vi "Run.vi"(8 "Column":i32, 9 "Row":i32, 10 "Maze (0: Empty, -1: Enemy. 1: Teammate)":i32[](array[numeric]), 11 "Line Dancer in":refnum<class "Brick Wall.lvclass">) -> (0 "Replicated":refnum<class "Square.lvclass">, 1 "Direction":T1, 2 "Action":T2, 3 "Line Dancer out":refnum<class "Brick Wall.lvclass">)   [LabVIEW 2015, in "Brick Wall.lvclass"]
uses:
  Brick Wall.lvclass
  Type Defs/Action Enum.ctl
  Type Defs/Direction Enum.ctl
  Square/Square.lvclass
  Common/Position.ctl
  Brick Wall.lvclass/Brick Wall.ctl
  Brick Wall Type.ctl
  SubVIs/Read-Only Globals.vi
  Common/Reverse Direction.vi
  Type Defs/SB Type Defs.lvlib
  Common/Common.lvlib
panel:
  # "NW\nN\nNE\nE\nSE\nS\nSW\nW"
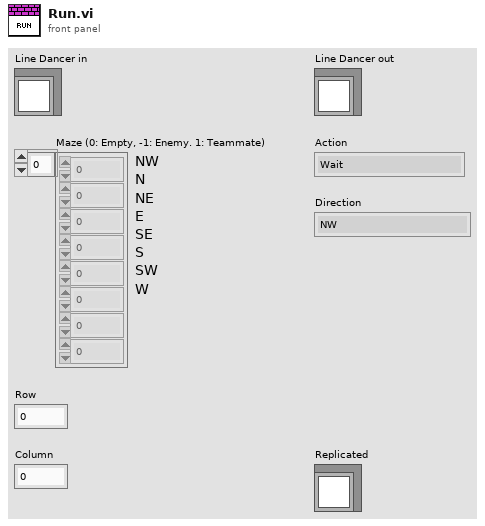
[diagram p1: front panel]
types:
  T1 = typedef "SB Type Defs.lvlib/Direction Enum.ctl" = enum16{"NW", "N", "NE", "E", "SE", "S", "SW", "W"}
  T2 = typedef "SB Type Defs.lvlib/Action Enum.ctl" = enum16{"Wait", "Move", "Attack", "Replicate"}
  T3 = typedef "Common.lvlib/Position.ctl" = cluster{"Column":i32, "Row":i32}
  T4 = typedef "Brick Wall.lvclass/Brick Wall Type.ctl" = enum16{"Row Starter", "Mover", "Starter", "Spawner", "Mason", "Wall"}
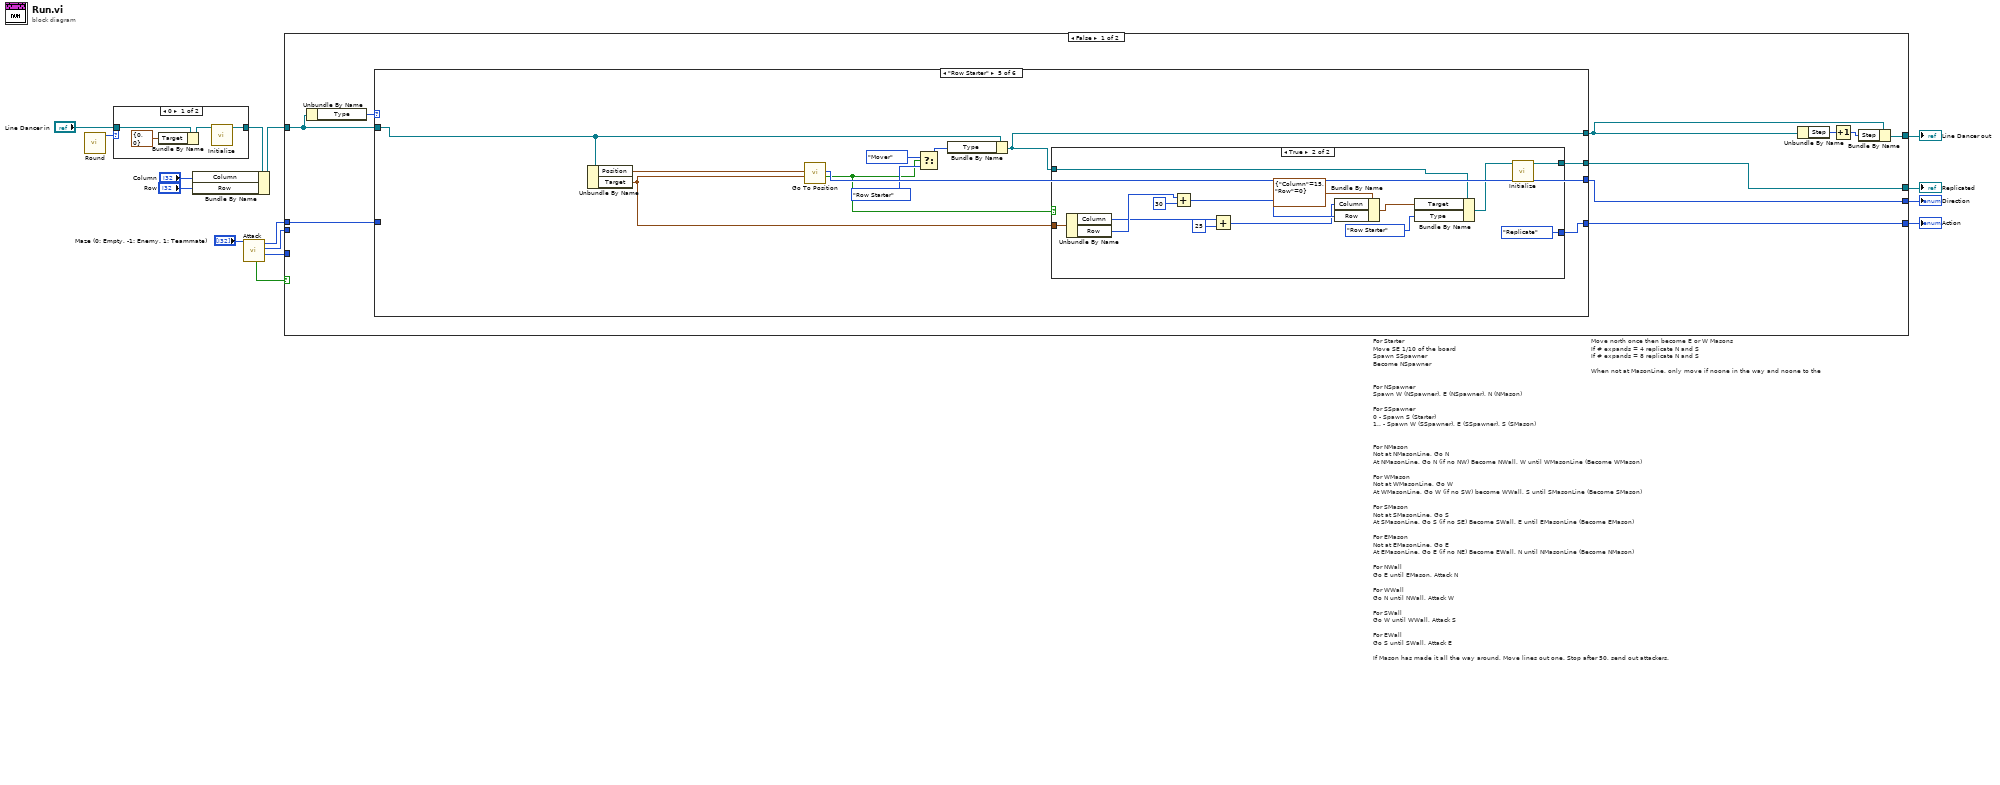
[diagram p0: block diagram]
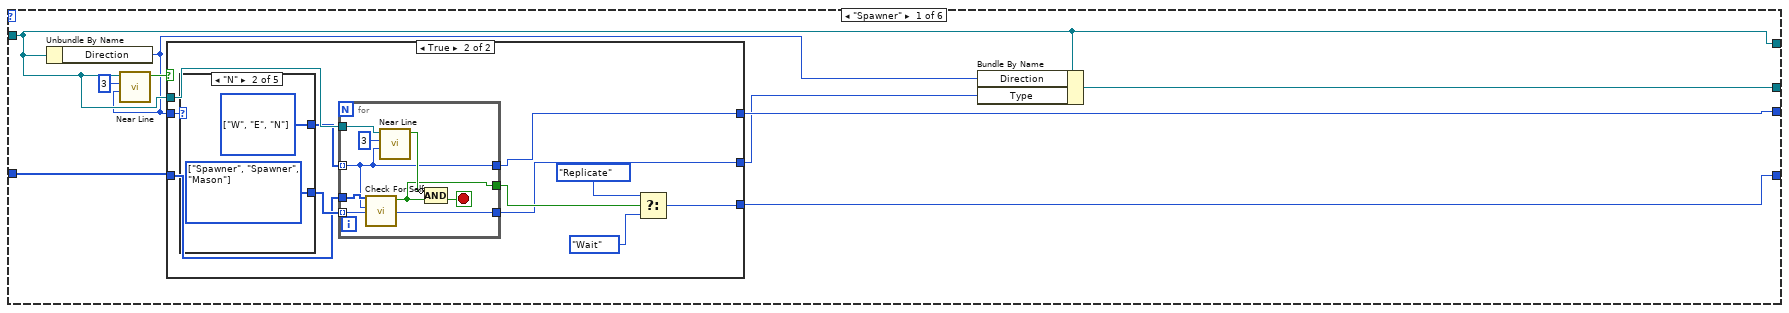
[diagram p2: hidden frame]
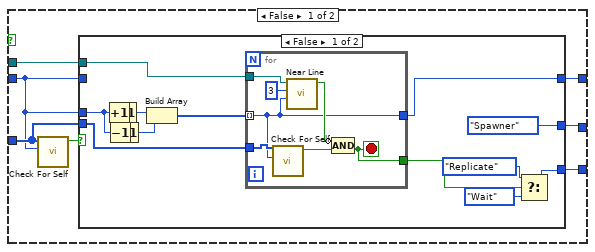
[diagram p3: hidden frame]
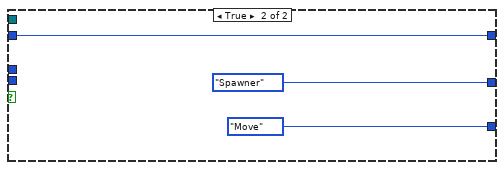
[diagram p4: hidden frame]
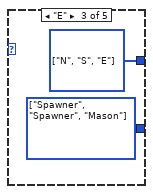
[diagram p6: hidden frame]
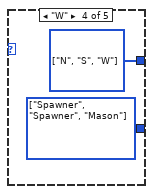
[diagram p7: hidden frame]
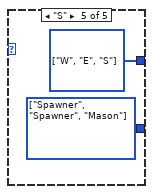
[diagram p8: hidden frame]
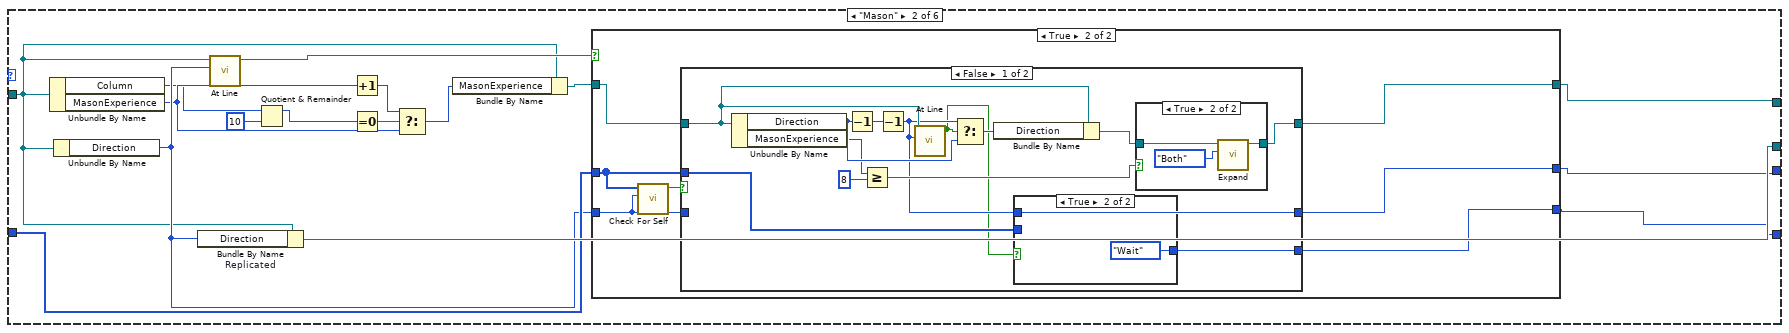
[diagram p9: hidden frame]
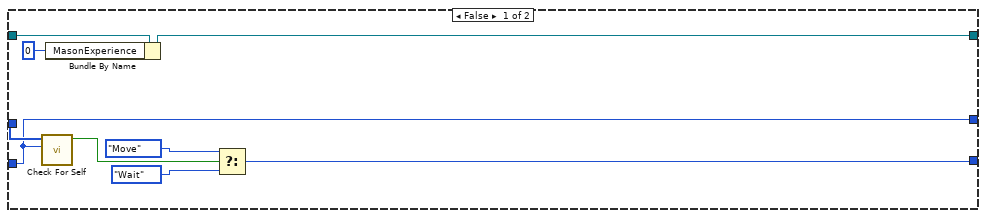
[diagram p10: hidden frame]
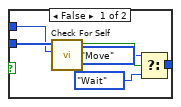
[diagram p11: hidden frame]
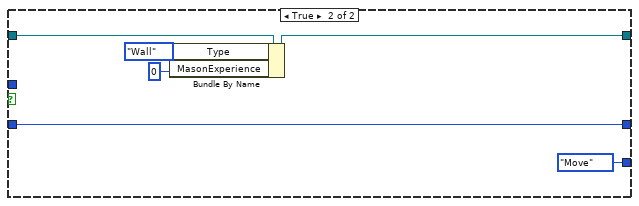
[diagram p13: hidden frame]
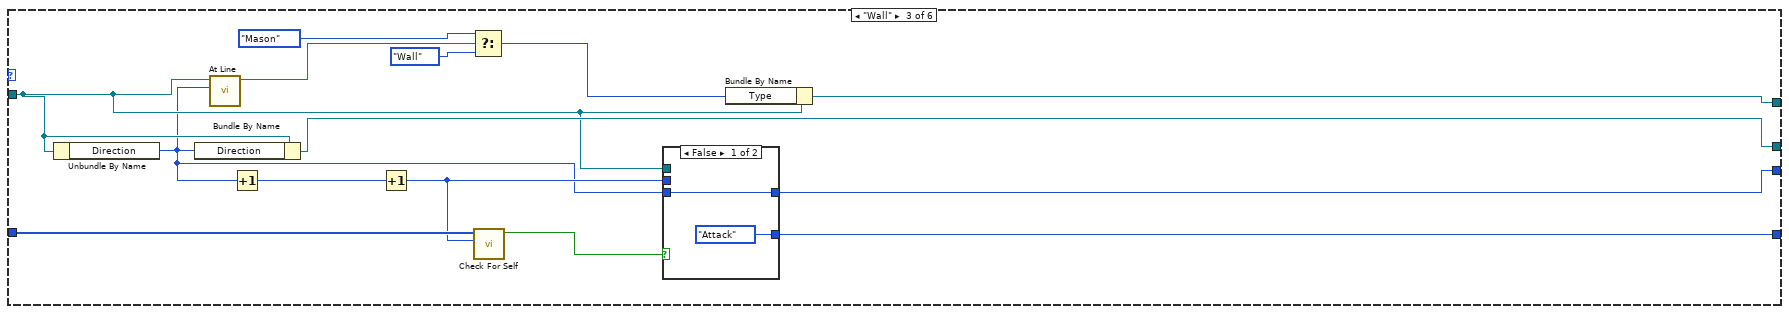
[diagram p14: hidden frame]
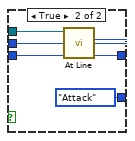
[diagram p15: hidden frame]
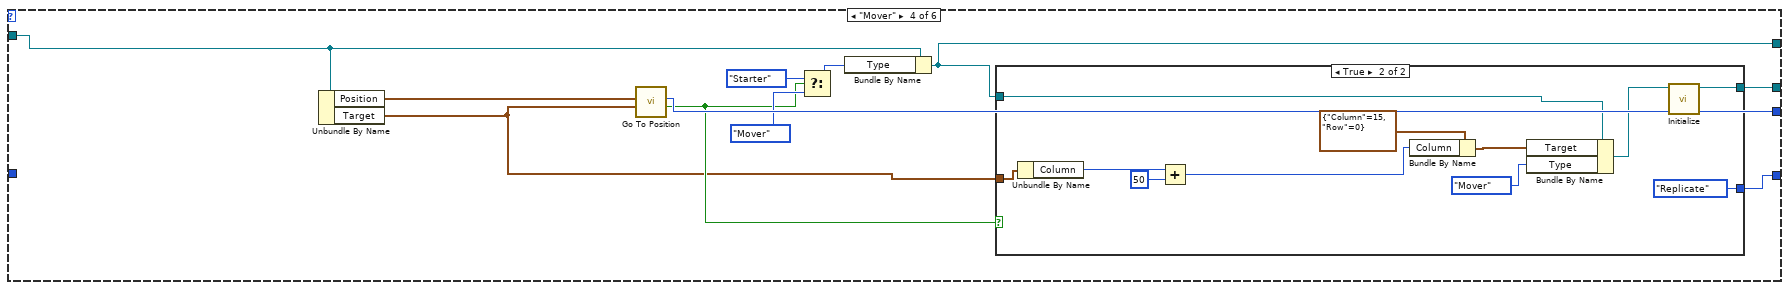
[diagram p16: hidden frame]
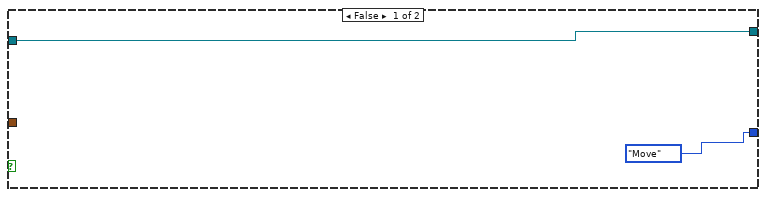
[diagram p17: hidden frame]
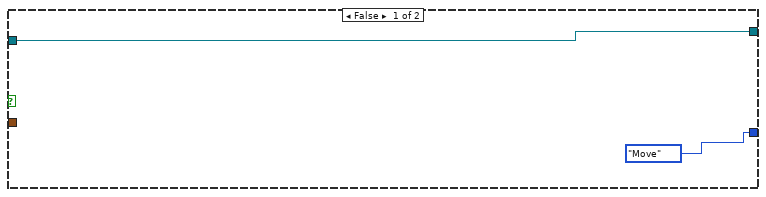
[diagram p18: hidden frame]
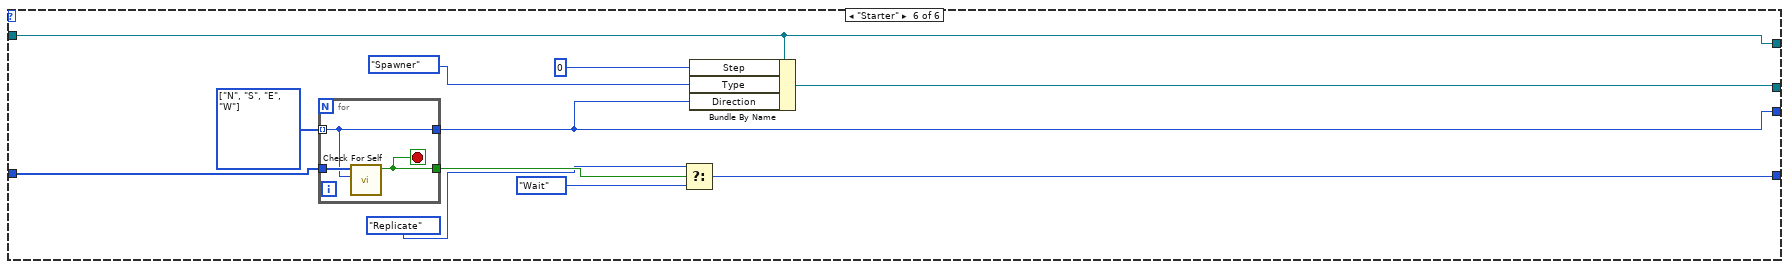
[diagram p19: hidden frame]
diagram:
  # "Move north once then become E or W Masons\nIf # expands = 4 replicate N and S\nIf # expands = 8 replicate N and S\n\nWhen not at MasonLine, only move if noone in the way and noone to the"
  # "For Starter \nMove SE 1/10 of the board\nSpawn SSpawner\nBecome NSpawner\n\n\nFor NSpawner\nSpawn W (NSpawner), E (NSpawner), N (NMason)\n\nFor SSpawner\n0 - Spawn S (Starter)\n1.. - Spawn W (SSpawner), E (SSpawner), S (SMason)\n\n\nFor NMason\nNot at NMasonLine, Go N\nAt NMasonLine, Go N (if no NW) Become NWall, W until WMasonLine (Become WMason)\n\nFor WMason\nNot at WMasonLine, Go W\nAt WMasonLine, Go W (if no SW) become WWall, S until SMasonLine (Become SMason)\n\nFor SMason\nNot at SMasonLine, Go S\nAt SMasonLine, Go S (if no SE) Become SWall, E until EMasonLine (Become EMason)\n\nFor EMason\nNot at EMasonLine, Go E\nAt EMasonLine, Go E (if no NE) Become EWall, N until NMasonLine (Become NMason)\n\nFor NWall\nGo E until EMason, Attack N\n\nFor WWall\nGo N until NWall, Attack W\n\nFor SWall\nGo W until WWall, Attack S\n\nFor EWall\nGo S until SWall, Attack E\n\nIf Mason has made it all the way around, Move lines out one. Stop after 50, send out attackers."
  n1 = call "Round.vi"() -> ("Round"=w5:i32)  [unwired: 11 in]
  n2 = case shown="0" w5 {
    tunnel: "Line Dancer in" -> [w19 w20]
    tunnel: [w18 w20] -> w6
    frame 0 {
      n3 = Bundle By Name(cluster=w19, "Target"=T3 {"Column"=0, "Row"=0}) -> (w17:refnum<class "Brick Wall.lvclass">)
      n4 = call "Initialize.vi"("Brick Wall in"=w17) -> ("Brick Wall out"=w18:refnum<class "Brick Wall.lvclass">)  [unwired: 10 in]
    }
    frame Default {
    }
  }
  n5 = Bundle By Name(cluster=w6, "Column"="Column", "Row"="Row") -> (w3:refnum<class "Brick Wall.lvclass">)
  n6 = call "Attack.vi"("Maze (0: Empty, -1: Enemy. >0: Teammate"="Maze (0: Empty, -1: Enemy. 1: Teammate)") -> ("Direction"=w8:i32, "Action"=w9:T2, "Maze (0: Empty, -1: Enemy. >0: Teammate 2"=w11:i32[], "Enemy Found?"=w10:bool)  [unwired: 5 in, 2 out]
  n7 = case shown="False" w10 {
    tunnel: [w24 w246] -> w15
    tunnel: [w23 w245] -> w14
    tunnel: w3 -> [w30 w247]
    tunnel: [w27 w247] -> w13
    tunnel: [w26 w247] -> w12
    tunnel: w11 -> [w22 _]
    tunnel: w9 -> [_ w246]
    tunnel: w8 -> [_ w245]
    frame False {
      n8 = Unbundle By Name(w30) -> ("Type"=w21:T4)
      n9 = case shown="\"Row Starter\"" w21 {
        tunnel: [w37 w101 w165 w181 w205 w237] -> w24
        tunnel: [w38 w102 w161 w190 w214 w231] -> w23
        tunnel: w22 -> [w39 w111 w164 _ _ w238]
        tunnel: [w36 w113 w173 w184 w208 w240] -> w26
        tunnel: [w32 w103 w171 w183 w207 w234] -> w25
        tunnel: w30 -> [w32 w105 w167 w186 w210 w234]
        frame "Spawner" {
          n10 = Unbundle By Name(w32) -> ("Direction"=w31:T1)
          n11 = call "Near Line.vi"("Line"=w31, "How Near?"=3, "Brick Wall in"=w32) -> ("Near Line"=w34:bool)  [unwired: 8 in]
          n12 = case shown="True" w34 {
            tunnel: w39 -> [w44 w71]
            tunnel: [w42 w72] -> w38
            tunnel: [w46 w81] -> w37
            tunnel: [w43 w73] -> w35
            tunnel: w31 -> [w41 w78]
            tunnel: w32 -> [w40 w77]
            frame False {
              n13 = call "Check For Self.vi"("Direction"=w41, "Map"=w44) -> ("Clear?"=w45:bool)  [unwired: 9 in]
              n14 = case shown="False" w45 {
                tunnel: [w50 Action_Enum."Move" ("f")] -> w46
                tunnel: w44 -> [w59 _]
                tunnel: [Brick_Wall_Type."Spawner" ("Player. Type") Brick_Wall_Type."Spawner" ("Player. Type")] -> w43
                tunnel: w41 -> [w56 _]
                tunnel: [w49 w69] -> w42
                tunnel: w41 -> [_ w69]
                tunnel: w40 -> [w47 _]
                frame False {
                  n15 = Increment(x=w56) -> (x+1=w58:T1)
                  n16 = Decrement(x=w56) -> (x-1=w57:T1)
                  n17 = Increment(x=w58) -> (x+1=w48:T1)
                  n18 = Decrement(x=w57) -> (x-1=w55:T1)
                  n19 = Build Array(w48, w55) -> (w54:T1[])
                  n20 = for {
                    tunnel: w54 -> [w61] mode=indexing
                    tunnel: [w61] -> w49
                    tunnel: [w63] -> w51
                    tunnel: w59 -> [w66]
                    tunnel: w47 -> [w64]
                    stop <- w63 stop-if-true
                    n21 = call "Check For Self.vi"("Direction"=w61, "Map"=w66) -> ("Clear?"=w67:bool)  [unwired: 9 in]
                    n22 = call "Near Line.vi"("Line"=w61, "How Near?"=3, "Brick Wall in"=w64) -> ("Near Line"=w62:bool)  [unwired: 8 in]
                    n23 = Compound Arithmetic op=AND(invert w62, w67) -> (w63:bool)
                  }
                  n24 = Select(t=Action_Enum."Replicate" ("f"), s=w51, f=Action_Enum."Wait") -> (s? t:f=w50:T2)
                }
                frame True {
                }
              }
            }
            frame True {
              n25 = case shown="\"N\"" w78 {
                tunnel: [_ w91 w93 w95 w97] -> w76
                tunnel: [_ w90 w92 w94 w96] -> w75
                frame Default {
                }
                frame "N" {
                  w90 = T4[] [enum."Spawner", enum."Spawner", enum."Mason"] items=["Row Starter", "Mover", "Starter", "Spawner", "Mason", "Wall"]
                  w91 = T1[] [enum."W", enum."E", enum."N"] items=["NW", "N", "NE", "E", "SE", "S", "SW", "W"]
                }
                frame "E" {
                  w92 = T4[] [enum."Spawner", enum."Spawner", enum."Mason"] items=["Row Starter", "Mover", "Starter", "Spawner", "Mason", "Wall"]
                  w93 = T1[] [enum."N", enum."S", enum."E"] items=["NW", "N", "NE", "E", "SE", "S", "SW", "W"]
                }
                frame "W" {
                  w94 = T4[] [enum."Spawner", enum."Spawner", enum."Mason"] items=["Row Starter", "Mover", "Starter", "Spawner", "Mason", "Wall"]
                  w95 = T1[] [enum."N", enum."S", enum."W"] items=["NW", "N", "NE", "E", "SE", "S", "SW", "W"]
                }
                frame "S" {
                  w96 = T4[] [enum."Spawner", enum."Spawner", enum."Mason"] items=["Row Starter", "Mover", "Starter", "Spawner", "Mason", "Wall"]
                  w97 = T1[] [enum."W", enum."E", enum."S"] items=["NW", "N", "NE", "E", "SE", "S", "SW", "W"]
                }
              }
              n26 = for {
                tunnel: w76 -> [w84] mode=indexing
                tunnel: [w84] -> w72
                tunnel: [w82] -> w74
                tunnel: w71 -> [w89]
                tunnel: w77 -> [w87]
                tunnel: w75 -> [w83] mode=indexing
                tunnel: [w83] -> w73
                stop <- w86 stop-if-true
                n27 = call "Check For Self.vi"("Direction"=w84, "Map"=w89) -> ("Clear?"=w82:bool)  [unwired: 9 in]
                n28 = call "Near Line.vi"("Line"=w84, "How Near?"=3, "Brick Wall in"=w87) -> ("Near Line"=w85:bool)  [unwired: 8 in]
                n29 = Compound Arithmetic op=AND(invert w85, w82) -> (w86:bool)
              }
              n30 = Select(t=Action_Enum."Replicate" ("f"), s=w74, f=Action_Enum."Wait") -> (s? t:f=w81:T2)
            }
          }
          n31 = Bundle By Name(cluster=w32, "Direction"=w31, "Type"=w35) -> (w36:refnum<class "Brick Wall.lvclass">)
        }
        frame "Mason" {
          n32 = Unbundle By Name(w105) -> ("Column"=w100:i32, "MasonExperience"=w107:u8)
          n33 = Unbundle By Name(w105) -> ("Direction"=w110:T1)
          n34 = Bundle By Name "Replicated"(cluster=w105, "Direction"=w110) -> (w113:refnum<class "Brick Wall.lvclass">)
          n35 = call "At Line.vi"("Line"=w110, "Brick Wall in"=w105) -> ("At Line"=w112:bool)  [unwired: 9 in]
          n36 = Quotient & Remainder(x=w100, y=10) -> (x-y*floor(x/y)=w99:i32)  [unwired: 1 out]
          n37 = Increment(x=w107) -> (x+1=w108:u8)
          n38 = Equal To 0?(x=w99) -> (x = 0?=w106:bool)
          n39 = Select(t=w108, s=w106, f=w107) -> (s? t:f=w109:u8)
          n40 = Bundle By Name(cluster=w105, "MasonExperience"=w109) -> (w104:refnum<class "Brick Wall.lvclass">)
          n41 = case shown="True" w112 {
            tunnel: [w116 w125] -> w101
            tunnel: [w117 w126] -> w102
            tunnel: w110 -> [w117 w124]
            tunnel: w111 -> [w118 w123]
            tunnel: w104 -> [w121 w129]
            tunnel: [w120 w127] -> w103
            frame False {
              n42 = call "Check For Self.vi"("Direction"=w117, "Map"=w118) -> ("Clear?"=w115:bool)  [unwired: 9 in]
              n43 = Bundle By Name(cluster=w121, "MasonExperience"=u8 0) -> (w120:refnum<class "Brick Wall.lvclass">)
              n44 = Select(t=Action_Enum."Move", s=w115, f=Action_Enum."Wait") -> (s? t:f=w116:T2)
            }
            frame True {
              n45 = call "Check For Self.vi"("Direction"=w124, "Map"=w123) -> ("Clear?"=w128:bool)  [unwired: 9 in]
              n46 = case shown="False" w128 {
                tunnel: [w135 w158] -> w127
                tunnel: w129 -> [w140 w159]
                tunnel: w124 -> [_ w156]
                tunnel: [w131 w156] -> w126
                tunnel: [w132 Action_Enum."Move" ("f")] -> w125
                tunnel: w123 -> [w133 _]
                frame False {
                  n47 = Unbundle By Name(w140) -> ("Direction"=w142:T1, "MasonExperience"=w138:u8)
                  n48 = Decrement(x=w142) -> (x-1=w141:T1)
                  n49 = Greater Or Equal?(x=w138, y=u8 8) -> (x >= y?=w134:bool)
                  n50 = Decrement(x=w141) -> (x-1=w131:T1)
                  n51 = call "At Line.vi"("Line"=w131, "Brick Wall in"=w140) -> ("At Line"=w130:bool)  [unwired: 9 in]
                  n52 = Select(t=w131, s=w130, f=w142) -> (s? t:f=w139:T1)
                  n53 = Bundle By Name(cluster=w140, "Direction"=w139) -> (w136:refnum<class "Brick Wall.lvclass">)
                  n54 = case shown="True" w130 {
                    tunnel: w133 -> [w148 _]
                    tunnel: [w144 Action_Enum."Wait" ("f")] -> w132
                    tunnel: w131 -> [w143 _]
                    frame False {
                      n55 = call "Check For Self.vi"("Direction"=w143, "Map"=w148) -> ("Clear?"=w146:bool)  [unwired: 9 in]
                      n56 = Select(t=Action_Enum."Move", s=w146, f=Action_Enum."Wait") -> (s? t:f=w144:T2)
                    }
                    frame True {
                    }
                  }
                  n57 = case shown="True" w134 {
                    tunnel: w136 -> [w150 w153]
                    tunnel: [w150 w152] -> w135
                    frame False {
                    }
                    frame True {
                      n58 = call-dynamic "Expand.vi"("Expand Direction"=enum16{"Height", "Width", "Both"}."Both", "Brick Wall in"=w153) -> ("Brick Wall out"=w152:refnum<class "Brick Wall.lvclass">)  [unwired: 8 in, 1 out]
                    }
                  }
                }
                frame True {
                  n59 = Bundle By Name(cluster=w159, "Type"=Brick_Wall_Type."Wall" ("Player. Type"), "MasonExperience"=u8 0) -> (w158:refnum<class "Brick Wall.lvclass">)
                }
              }
            }
          }
        }
        frame "Wall" {
          n60 = Unbundle By Name(w167) -> ("Direction"=w160:T1)
          n61 = Bundle By Name(cluster=w167, "Direction"=w160) -> (w173:refnum<class "Brick Wall.lvclass">)
          n62 = call "At Line.vi"("Line"=w160, "Brick Wall in"=w167) -> ("At Line"=w172:bool)  [unwired: 9 in]
          n63 = Increment(x=w160) -> (x+1=w166:T1)
          n64 = Increment(x=w166) -> (x+1=w163:T1)
          n65 = Select(t=Brick_Wall_Type."Mason" ("Player. Type"), s=w172, f=Brick_Wall_Type."Wall" ("Player. Type")) -> (s? t:f=w168:T4)
          n66 = call "Check For Self.vi"("Direction"=w163, "Map"=w164) -> ("Clear?"=w162:bool)  [unwired: 9 in]
          n67 = case shown="False" w162 {
            tunnel: w167 -> [_ w179]
            tunnel: [Action_Enum."Attack" ("f") Action_Enum."Attack" ("f")] -> w165
            tunnel: w163 -> [_ w177]
            tunnel: [w174 w178] -> w161
            tunnel: w160 -> [w174 w178]
            frame False {
            }
            frame True {
              n68 = call "At Line.vi"("Line"=w177, "Brick Wall in"=w179) -> ()  [unwired: 9 in, 1 out]
            }
          }
          n69 = Bundle By Name(cluster=w167, "Type"=w168) -> (w171:refnum<class "Brick Wall.lvclass">)
        }
        frame "Mover" {
          n70 = Unbundle By Name(w186) -> ("Position"=w185:T3, "Target"=w180:T3)
          n71 = call "Go To Position.vi"("Target Position"=w180, "My Position"=w185) -> ("Arrived?"=w182:bool, "Direction"=w190:T1)  [unwired: 7 in, 1 out]
          n72 = Select(t=Brick_Wall_Type."Starter", s=w182, f=Brick_Wall_Type."Mover" ("Player. Type")) -> (s? t:f=w188:T4)
          n73 = Bundle By Name(cluster=w186, "Type"=w188) -> (w183:refnum<class "Brick Wall.lvclass">)
          n74 = case shown="True" w182 {
            tunnel: [w192 w193] -> w184
            tunnel: w183 -> [w192 w195]
            tunnel: [Action_Enum."Move" ("f") Action_Enum."Replicate" ("f")] -> w181
            tunnel: w180 -> [_ w196]
            frame False {
            }
            frame True {
              n75 = Unbundle By Name(w196) -> ("Column"=w199:i32)
              n76 = Add(x=w199, y=50) -> (x+y=w202:i32)
              n77 = Bundle By Name(cluster=T3 {"Column"=15, "Row"=0} ("Target"), "Column"=w202) -> (w201:T3)
              n78 = Bundle By Name(cluster=w195, "Target"=w201, "Type"=Brick_Wall_Type."Mover" ("Player. Type")) -> (w194:refnum<class "Brick Wall.lvclass">)
              n79 = call "Initialize.vi"("Brick Wall in"=w194) -> ("Brick Wall out"=w193:refnum<class "Brick Wall.lvclass">)  [unwired: 10 in]
            }
          }
        }
        frame "Row Starter" {
          n80 = Unbundle By Name(w210) -> ("Position"=w209:T3, "Target"=w204:T3)
          n81 = call "Go To Position.vi"("Target Position"=w204, "My Position"=w209) -> ("Arrived?"=w206:bool, "Direction"=w214:T1)  [unwired: 7 in, 1 out]
          n82 = Select(t=Brick_Wall_Type."Mover", s=w206, f=Brick_Wall_Type."Row Starter" ("Player. Type")) -> (s? t:f=w212:T4)
          n83 = Bundle By Name(cluster=w210, "Type"=w212) -> (w207:refnum<class "Brick Wall.lvclass">)
          n84 = case shown="True" w206 {
            tunnel: [w216 w217] -> w208
            tunnel: w207 -> [w216 w219]
            tunnel: [Action_Enum."Move" ("f") Action_Enum."Replicate" ("f")] -> w205
            tunnel: w204 -> [_ w220]
            frame False {
            }
            frame True {
              n85 = Unbundle By Name(w220) -> ("Column"=w223:i32, "Row"=w228:i32)
              n86 = Add(x=w228, y=30) -> (x+y=w229:i32)
              n87 = Add(x=w223, y=25) -> (x+y=w226:i32)
              n88 = Bundle By Name(cluster=T3 {"Column"=15, "Row"=0} ("Target"), "Column"=w226, "Row"=w229) -> (w225:T3)
              n89 = Bundle By Name(cluster=w219, "Target"=w225, "Type"=Brick_Wall_Type."Row Starter" ("Player. Type")) -> (w218:refnum<class "Brick Wall.lvclass">)
              n90 = call "Initialize.vi"("Brick Wall in"=w218) -> ("Brick Wall out"=w217:refnum<class "Brick Wall.lvclass">)  [unwired: 10 in]
            }
          }
        }
        frame "Starter" {
          w232 = T1[] [enum."N", enum."S", enum."E", enum."W"] items=["NW", "N", "NE", "E", "SE", "S", "SW", "W"]
          n91 = for {
            tunnel: w238 -> [w244]
            tunnel: w232 -> [w242] mode=indexing
            tunnel: [w243] -> w236
            tunnel: [w242] -> w231
            stop <- w243 stop-if-true
            n92 = call "Check For Self.vi"("Direction"=w242, "Map"=w244) -> ("Clear?"=w243:bool)  [unwired: 9 in]
          }
          n93 = Select(t=Action_Enum."Replicate", s=w236, f=Action_Enum."Wait") -> (s? t:f=w237:T2)
          n94 = Bundle By Name(cluster=w234, "Step"=0, "Type"=Brick_Wall_Type."Spawner" ("Player Type"), "Direction"=w231) -> (w240:refnum<class "Brick Wall.lvclass">)
        }
      }
      n95 = Unbundle By Name(w25) -> ("Step"=w29:i32)
      n96 = Increment(x=w29) -> (x+1=w28:i32)
      n97 = Bundle By Name(cluster=w25, "Step"=w28) -> (w27:refnum<class "Brick Wall.lvclass">)
    }
    frame True {
    }
  }
  "Line Dancer out" <- w13
  "Action" <- w15
  "Direction" <- w14
  "Replicated" <- w12
